vi "CLC_L1_ParsingData.vi"() -> ()   [LabVIEW 2023, in "Clover_Cell.lvlib"]
uses:
  <vilib>/Utility/file.llb/Read Delimited Spreadsheet (string).vi
  Clover_Cell.lvlib
panel:
  out "Array":dbl[][](array[numeric])
  out "Waveform Graph":dbl[][](graph)
  out "subarray":string[](array[string])
  in  "Function":T1(ring)
  out "element":string
  in  "Test Item":u16(ring) items=["TX_H_Ch0_Freq26.5_In_Phase_Step", "TX_H_Ch0_Freq28_In_Phase_Step", "TX_H_Ch0_Freq29.5_In_Phase_Step", "TX_H_Ch0_Freq31_In_Phase_Step", "TX_H_Ch1_Freq26.5_In_Phase_Step", "TX_H_Ch1_Freq28_In_Phase_Step", "TX_H_Ch1_Freq29.5_In_Phase_Step", "TX_H_Ch1_Freq31_In_Phase_Step", "TX_H_Ch2_Freq26.5_In_Phase_Step", "TX_H_Ch2_Freq28_In_Phase_Step", "TX_H_Ch2_Freq29.5_In_Phase_Step", "TX_H_Ch2_Freq31_In_Phase_Step", "TX_H_Ch3_Freq26.5_In_Phase_Step", "TX_H_Ch3_Freq28_In_Phase_Step", "TX_H_Ch3_Freq29.5_In_Phase_Step", "TX_H_Ch3_Freq31_In_Phase_Step", "TX_V_Ch0_Freq26.5_In_Phase_Step", "TX_V_Ch0_Freq28_In_Phase_Step", "TX_V_Ch0_Freq29.5_In_Phase_Step", "TX_V_Ch0_Freq31_In_Phase_Step", "TX_V_Ch1_Freq26.5_In_Phase_Step", "TX_V_Ch1_Freq28_In_Phase_Step", "TX_V_Ch1_Freq29.5_In_Phase_Step", "TX_V_Ch1_Freq31_In_Phase_Step", "TX_V_Ch2_Freq26.5_In_Phase_Step", "TX_V_Ch2_Freq28_In_Phase_Step", "TX_V_Ch2_Freq29.5_In_Phase_Step", "TX_V_Ch2_Freq31_In_Phase_Step", "TX_V_Ch3_Freq26.5_In_Phase_Step", "TX_V_Ch3_Freq28_In_Phase_Step", "TX_V_Ch3_Freq29.5_In_Phase_Step", "TX_V_Ch3_Freq31_In_Phase_Step", "RX_H_Ch0_Freq26.5_In_Phase_Step", "RX_H_Ch0_Freq28_In_Phase_Step", "RX_H_Ch0_Freq29.5_In_Phase_Step", "RX_H_Ch0_Freq31_In_Phase_Step", "RX_H_Ch1_Freq26.5_In_Phase_Step", "RX_H_Ch1_Freq28_In_Phase_Step", "RX_H_Ch1_Freq29.5_In_Phase_Step", "RX_H_Ch1_Freq31_In_Phase_Step", "RX_H_Ch2_Freq26.5_In_Phase_Step", "RX_H_Ch2_Freq28_In_Phase_Step", "RX_H_Ch2_Freq29.5_In_Phase_Step", "RX_H_Ch2_Freq31_In_Phase_Step", "RX_H_Ch3_Freq26.5_In_Phase_Step", "RX_H_Ch3_Freq28_In_Phase_Step", "RX_H_Ch3_Freq29.5_In_Phase_Step", "RX_H_Ch3_Freq31_In_Phase_Step", "RX_V_Ch0_Freq26.5_In_Phase_Step", "RX_V_Ch0_Freq28_In_Phase_Step", "RX_V_Ch0_Freq29.5_In_Phase_Step", "RX_V_Ch0_Freq31_In_Phase_Step", "RX_V_Ch1_Freq26.5_In_Phase_Step", "RX_V_Ch1_Freq28_In_Phase_Step", "RX_V_Ch1_Freq29.5_In_Phase_Step", "RX_V_Ch1_Freq31_In_Phase_Step", "RX_V_Ch2_Freq26.5_In_Phase_Step", "RX_V_Ch2_Freq28_In_Phase_Step", "RX_V_Ch2_Freq29.5_In_Phase_Step", "RX_V_Ch2_Freq31_In_Phase_Step", "RX_V_Ch3_Freq26.5_In_Phase_Step", "RX_V_Ch3_Freq28_In_Phase_Step", "RX_V_Ch3_Freq29.5_In_Phase_Step", "RX_V_Ch3_Freq31_In_Phase_Step", "TX_H_com_gain_26.5GHz", "TX_V_com_gain_26.5GHz", "TX_H_com_gain_28GHz", "TX_V_com_gain_28GHz", "TX_H_com_gain_29.5GHz", "TX_V_com_gain_29.5GHz", "TX_H_com_gain_31GHz", "TX_V_com_gain_31GHz", "RX_H_com_gain_26.5GHz", "RX_V_com_gain_26.5GHz", "RX_H_com_gain_28GHz", "RX_V_com_gain_28GHz", "RX_H_com_gain_29.5GHz", "RX_V_com_gain_29.5GHz", "RX_H_com_gain_31GHz", "RX_V_com_gain_31GHz", "TX_H_all_gain_26.5GHz", "TX_V_all_gain_26.5GHz", "TX_H_all_gain_28GHz", "TX_V_all_gain_28GHz", "TX_H_all_gain_29.5GHz", "TX_V_all_gain_29.5GHz", "TX_H_all_gain_31GHz", "TX_V_all_gain_31GHz", "RX_H_all_gain_26.5GHz", "RX_V_all_gain_26.5GHz", "RX_H_all_gain_28GHz", "RX_V_all_gain_28GHz", "RX_H_all_gain_29.5GHz", "RX_V_all_gain_29.5GHz", "RX_H_all_gain_31GHz", "RX_V_all_gain_31GHz"]
  out "all rows":string[][](array[string])
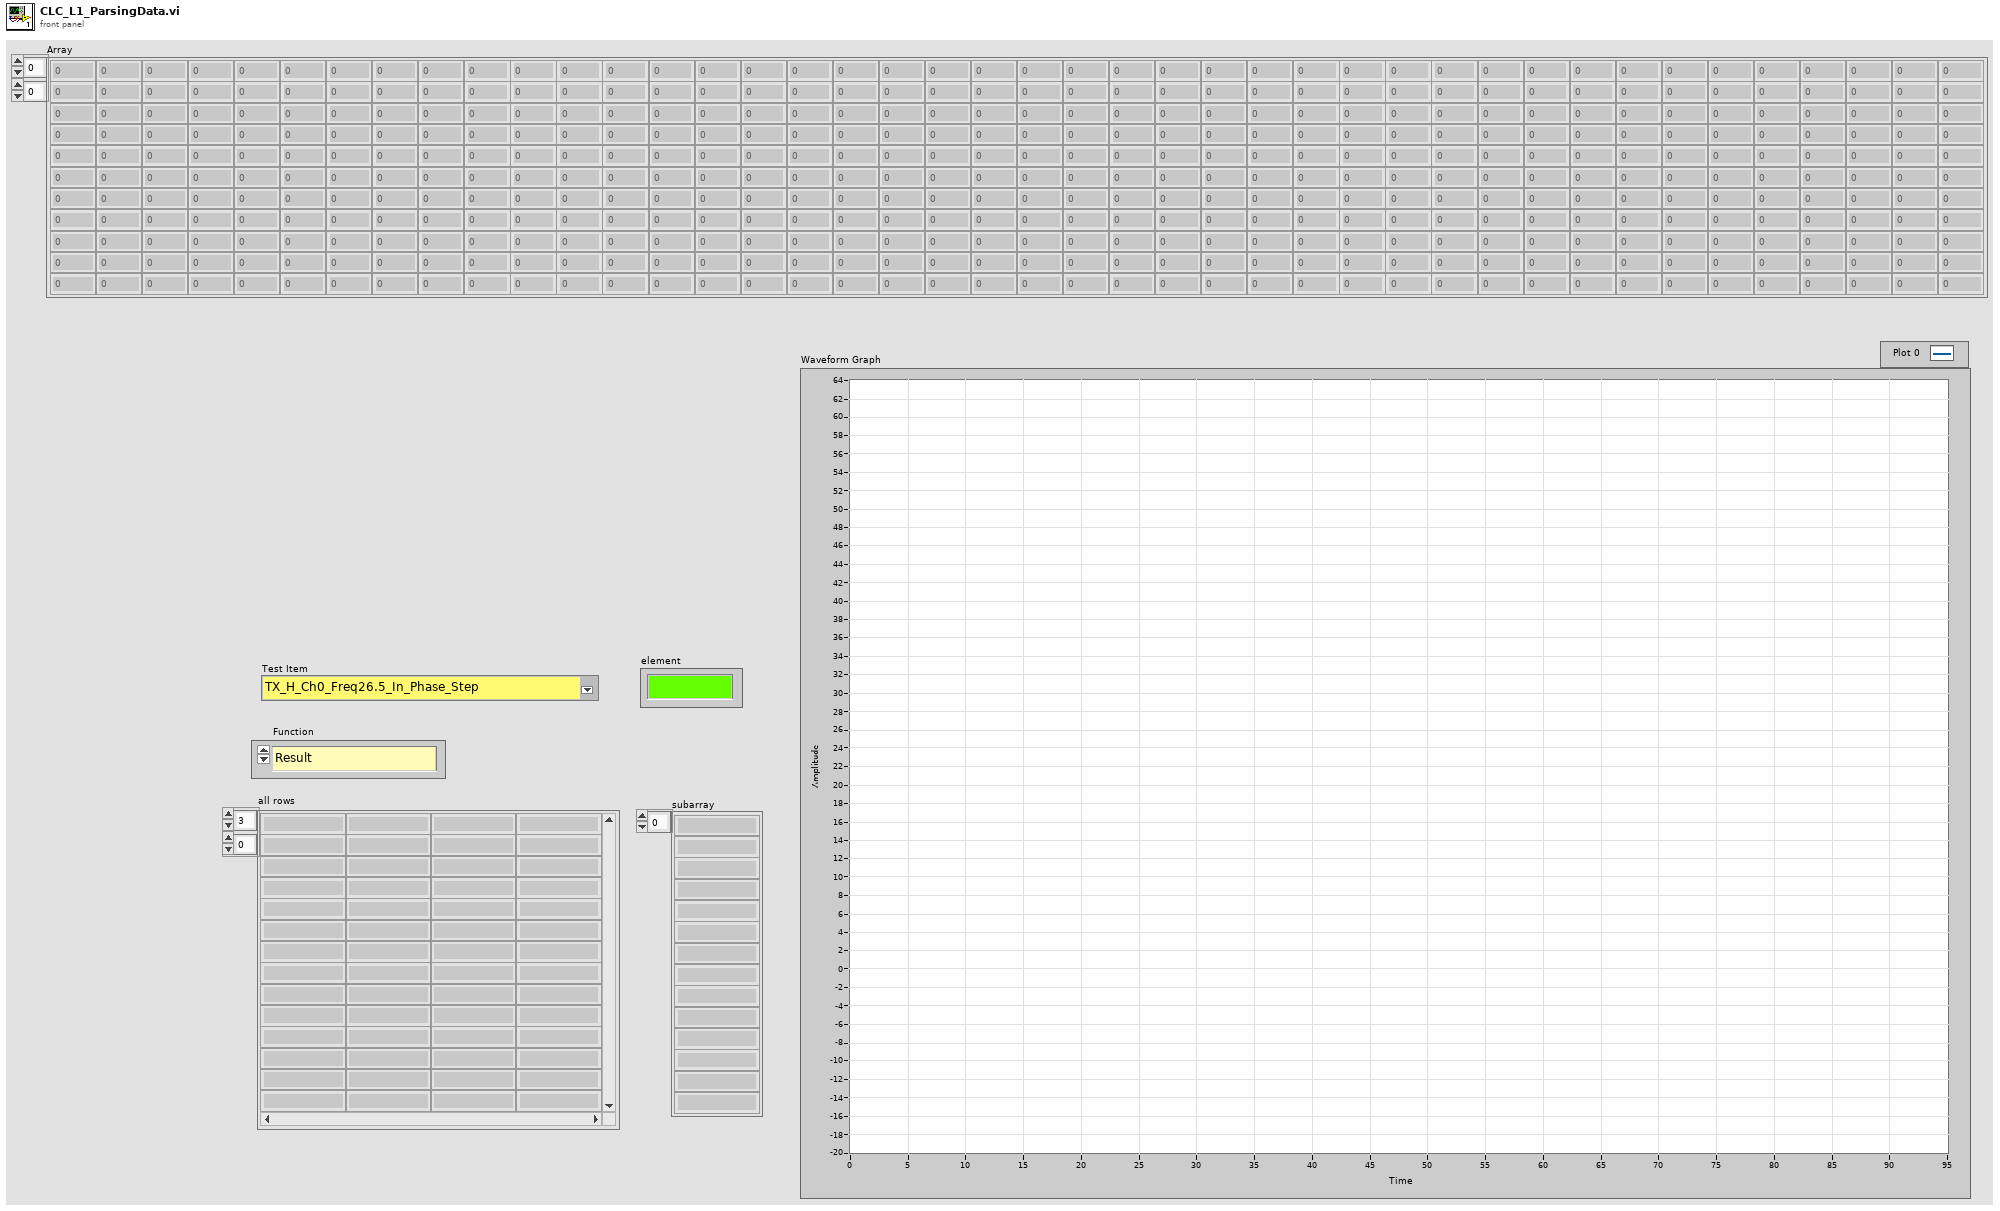
[diagram p1: front panel]
types:
  T1 = enum16{"Result", "Marker_1_26.5GHz", "Marker_2_28GHz", "Marker_3_29.5GHz", "Marker_4_31GHz"}
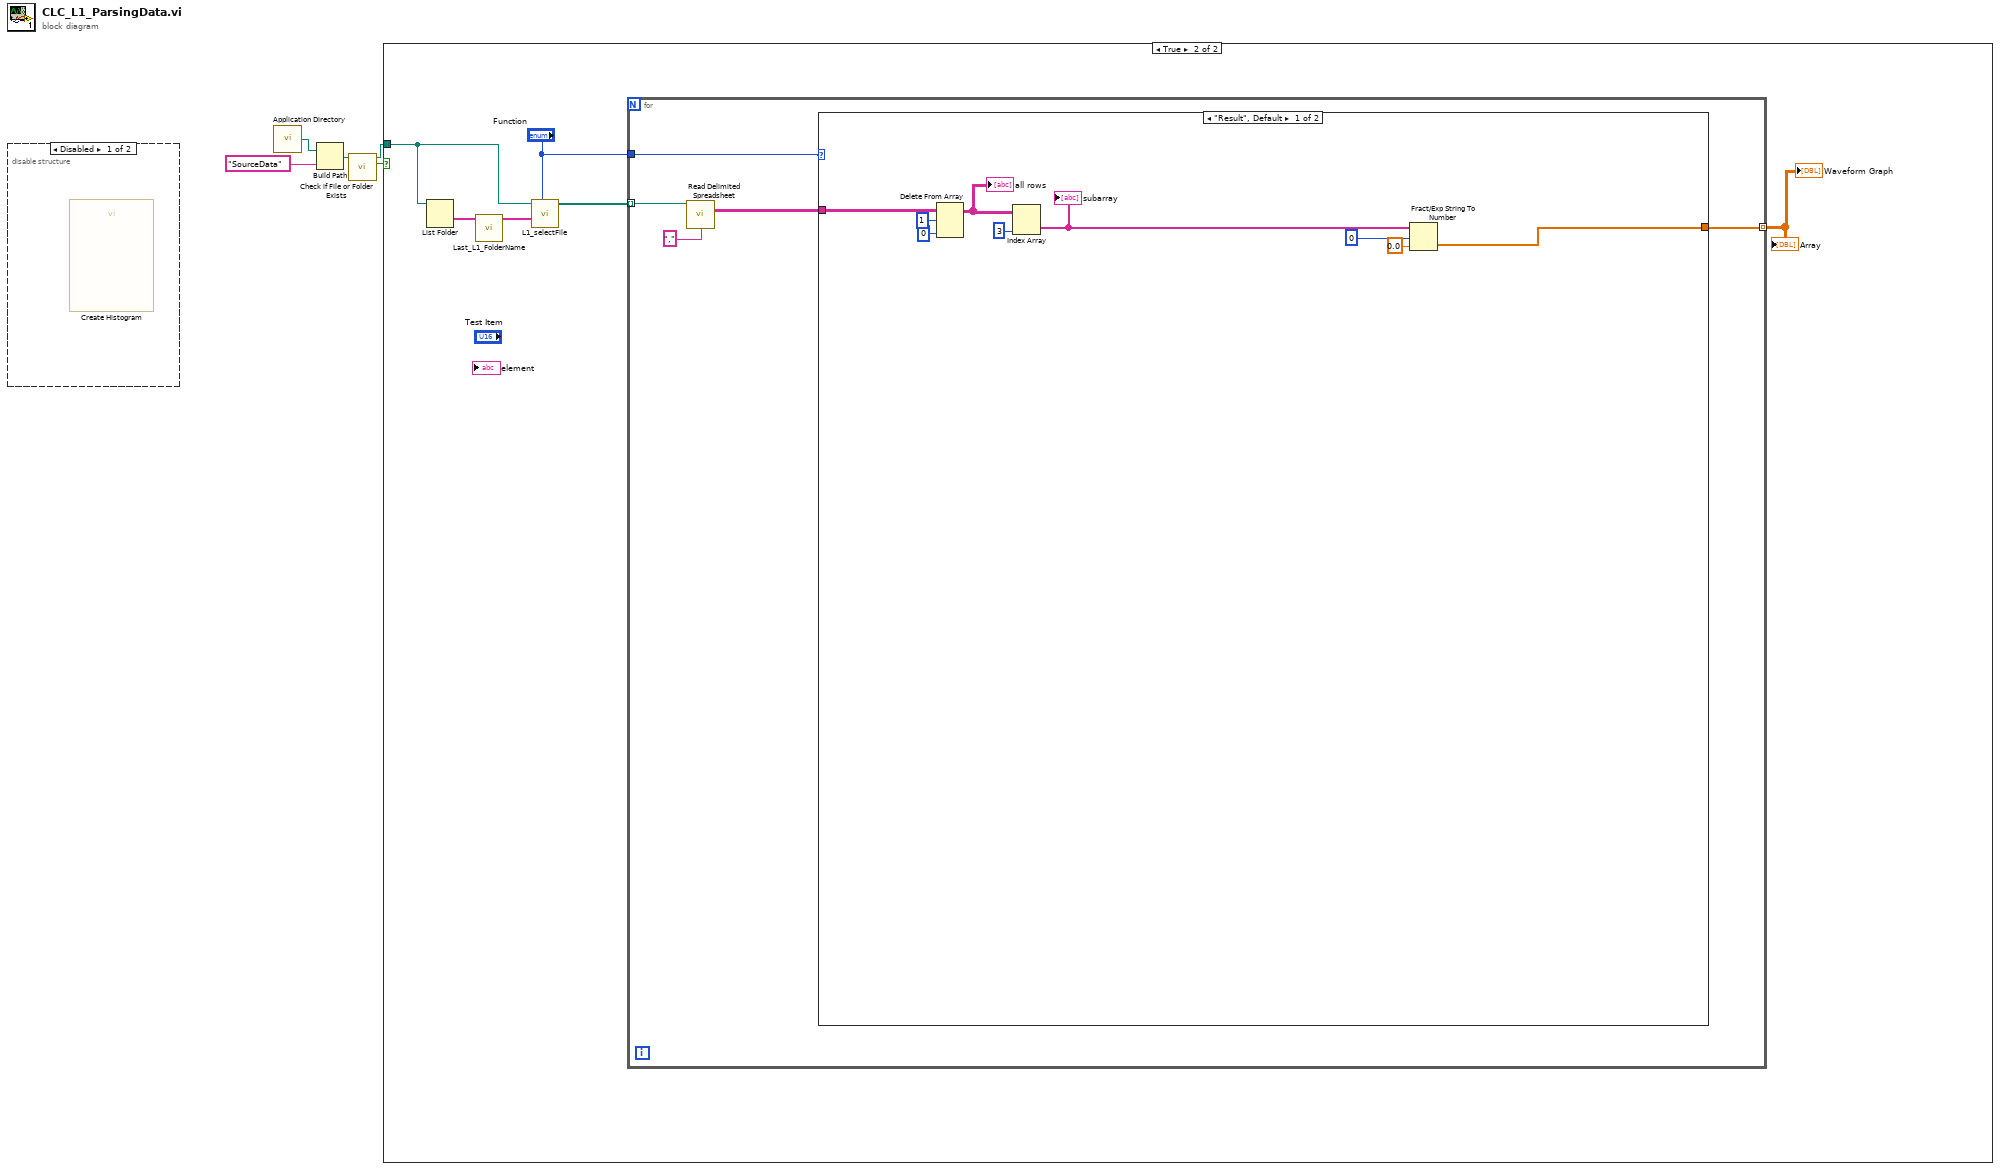
[diagram p0: block diagram]
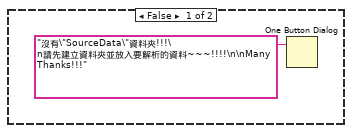
[diagram p3: hidden frame]
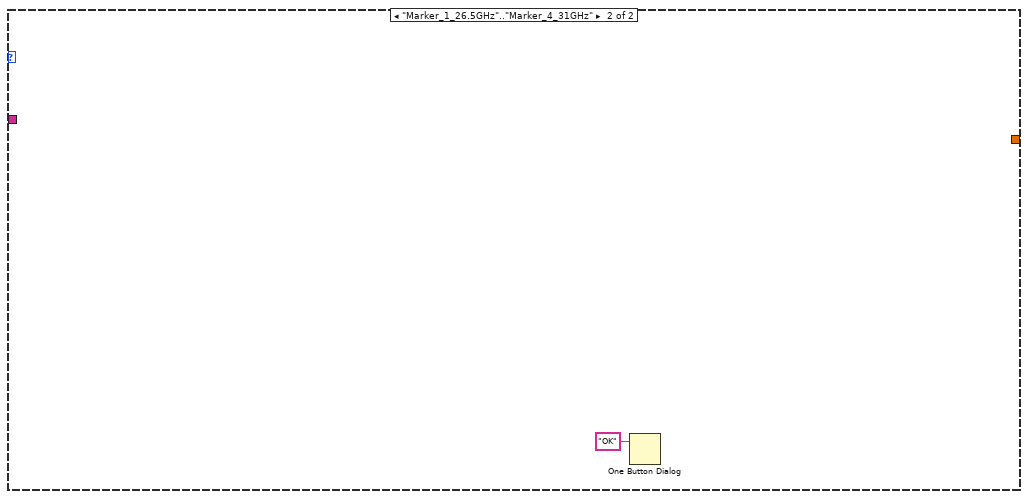
[diagram p4: hidden frame]
diagram:
  n1 = disable-structure shown="Disabled" {
    frame Disabled {
      n2 = call "Create Histogram"() -> ()  [unwired: 10 in, 2 out]
    }
    frame Enabled {
    }
  }
  n3 = call <vilib>:"Application Directory.vi"() -> ("Application Directory"=w4:path)
  n4 = Build Path(base path=w4, name or relative path="SourceData") -> (appended path=w1:path)
  n5 = call <vilib>:"Check if File or Folder Exists.vi"("path"=w1) -> ("file or folder exists?"=w3:bool, "dup path"=w2:path)  [unwired: 8 in, 1 out]
  n6 = case shown="True" w3 {
    tunnel: w2 -> [_ w10]
    frame False {
      n7 = One Button Dialog(message="沒有\"SourceData\"資料夾!!!\n請先建立資料夾並放入要解析的資料~~~!!!!\n\nMany Thanks!!!") -> ()  [unwired: 1 in, 1 out]
    }
    frame True {
      n8 = List Folder(path=w10) -> (folder names=w12:string[])  [unwired: 3 in, 3 out]
      n9 = call "Last_L1_FolderName.vi"("folder names"=w12) -> ("File_Name"=w11:string[])  [unwired: 10 in]
      n10 = call "L1_selectFile.vi"("Function"="Function", "File_Name"=w11, "dup path"=w10) -> ("FileName_path"=w9:path[])  [unwired: 7 in, 1 out]
      n11 = for {
        tunnel: w9 -> [w16] mode=indexing
        tunnel: "Function" -> [w15]
        tunnel: [w13] -> w7 mode=indexing
        n12 = call-poly <vilib>:"Read Delimited Spreadsheet.vi"("file path (dialog if empty)"=w16, "delimiter (\\t)"="," ("delimiter (\\t)")) -> ("all rows"=w14:string[][])  [unwired: 8 in, 5 out]
        n13 = case shown="\"Result\", Default" w15 {
          tunnel: w14 -> [w26 _]
          tunnel: [w19 _] -> w13
          frame "Result", Default {
            n14 = Delete From Array(array=w26, length=1, index (row)=0) -> (array with subset deleted=w23:string[][])  [unwired: 1 in, 1 out]
            "all rows" <- w23
            n15 = Index Array(array=w23, index (col)=3 ("disabled index (col)")) -> (element=w21:string[])  [unwired: 1 in]
            "subarray" <- w21
            n16 = Fract/Exp String To Number(string=w21, offset=0, default (0 dbl)=0.0 ("default (0 DBL)")) -> (number=w19:dbl[])  [unwired: 1 in, 1 out]
          }
          frame "Marker_1_26.5GHz".."Marker_4_31GHz" {
            n17 = One Button Dialog(message="OK") -> ()  [unwired: 1 in, 1 out]
          }
        }
      }
      "Waveform Graph" <- w7
      "Array" <- w7
    }
  }
